vi "attribute_get_cache_or_default_value.vi"(7 "Attribute":T1={"Identifier"="", "Descriptive name"="", "Data Type"=enum."Integer 32", "Command"="", "Access"=2, "Range Table"="", "Read Callback"="", "Write Callback"="", "Range Callback"="", "Check Callback"="", "Rngtable Callback"="", "Coerce Callback"="", "Supported Models"="", "Instrument Options"="", "Repeated Capabilities"="", "Check Status Callback"="", "Index"=0, "Flag: OPC Wait"=FALSE, "Flag: Dont check status"=FALSE, "Flag: Cache Only"=FALSE} {"Access" items=["Read Only", "Write Only", "Read/Write"]}, 8 "error in":errorcluster, 11 "VISA resource name":refnum<visa-resource-name>) -> (0 "error out":errorcluster, 1 "Integer 32 out":i32, 2 "Double out":dbl, 3 "VISA resource name out":refnum<visa-resource-name>, 4 "String out":string, 5 "Integer 64 out":i64, 6 "Boolean out":bool, 9 "Exists in cache":bool)   [LabVIEW 2014, in "rszvl_rsidr_core.lvlib"]
uses:
  rszvl_rsidr_core.lvlib
  type_Attribute.ctl
  type_Attribute_Data_Type.ctl
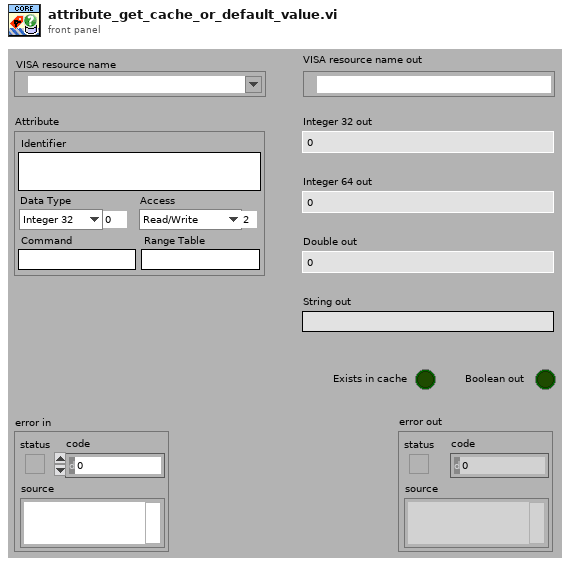
[diagram p1: front panel]
types:
  T1 = typedef "rszvl_rsidr_core.lvlib/type_Attribute.ctl" = cluster{"Identifier":string, "Descriptive name":string, "Data Type":T2, "Command":string, "Access":u16, "Range Table":string, "Read Callback":string, "Write Callback":string, "Range Callback":string, "Check Callback":string, "Rngtable Callback":string, "Coerce Callback":string, "Supported Models":string, "Instrument Options":string, "Repeated Capabilities":string, "Check Status Callback":string, "Index":i32, "Flag: OPC Wait":bool, "Flag: Dont check status":bool, "Flag: Cache Only":bool}
  T2 = typedef "rszvl_rsidr_core.lvlib/type_Attribute_Data_Type.ctl" = enum16{"Integer 32", "Double", "String", "Boolean", "None", "Integer 64"}
  T3 = enum16{"Initialize", "Check", "Get Numeric Value", "Get Default Value"}
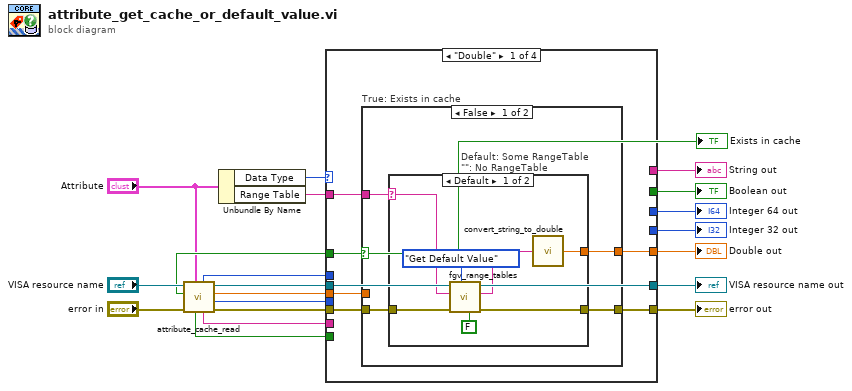
[diagram p0: block diagram]
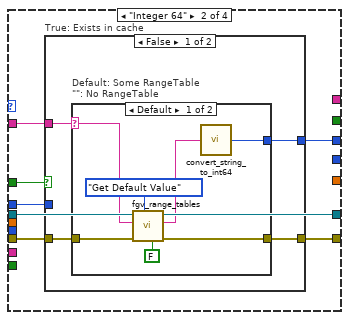
[diagram p4: hidden frame]
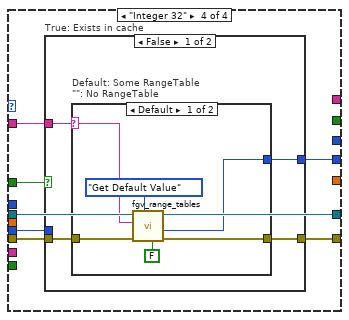
[diagram p8: hidden frame]
diagram:
  n1 = call "attribute_cache_read.vi"("Attribute"="Attribute", "error in"="error in", "VISA resource name"="VISA resource name") -> ("error out"=w12:errorcluster, "Integer 32 out"=w6:i32, "Double out"=w9:dbl, "VISA resource name out"=w11:refnum<visa-resource-name>, "String out"=w5:string, "Integer 64 out"=w8:i64, "Boolean out"=w3:bool, "Exists in cache"=w10:bool)  [unwired: 1 in]
  "Exists in cache" <- w10
  n2 = Unbundle By Name("Attribute") -> ("Data Type"=w17:T2, "Range Table"=w7:string)
  n3 = case shown="\"Double\"" w17 {
    tunnel: w12 -> [w24 w43 w66 w69]
    tunnel: w11 -> [w25 w44 w65 w70]
    tunnel: [w27 w48 w66 w73] -> w20
    tunnel: [w25 w44 w65 w70] -> w19
    tunnel: [w26 _ _ _] -> w18
    tunnel: [_ _ _ w72] -> w16
    tunnel: [_ w47 _ _] -> w15
    tunnel: w10 -> [w22 w45 _ w67]
    tunnel: w9 -> [w23 _ _ _]
    tunnel: w8 -> [_ w46 _ _]
    tunnel: w7 -> [w21 w42 _ w71]
    tunnel: w6 -> [_ _ _ w68]
    tunnel: w5 -> [_ _ w64 _]
    tunnel: [_ _ w64 _] -> w4
    tunnel: w3 -> [_ _ w63 _]
    tunnel: [_ _ w63 _] -> w2
    frame "Double" {
      n4 = case "True: Exists in cache" shown="False" w22 {
        tunnel: w24 -> [w30 w41]
        tunnel: w23 -> [_ w40]
        tunnel: [w29 w41] -> w27
        tunnel: w21 -> [w31 _]
        tunnel: [w28 w40] -> w26
        frame False {
          n5 = case "Default: Some RangeTable\n\"\": No RangeTable" shown="Default" w31 {
            selector: w31 -> [w35 _]
            tunnel: w30 -> [w38 w39]
            tunnel: [w37 w39] -> w29
            tunnel: [w33 _] -> w28
            frame Default {
              n6 = call "fgv_range_tables.vi"("Range Checking"=FALSE, "Operation"=T3."Get Default Value", "error in"=w38, "Range Table ID in"=w35) -> ("error out"=w37:errorcluster, "Default value out"=w32:string)  [unwired: 4 in, 2 out]
              n7 = call "convert_string_to_double.vi"("String in"=w32) -> ("double value out"=w33:dbl)  [unwired: 4 in]
            }
            frame "" {
            }
          }
        }
        frame True {
        }
      }
    }
    frame "Integer 64" {
      n8 = case "True: Exists in cache" shown="False" w45 {
        tunnel: w43 -> [w51 w62]
        tunnel: w46 -> [_ w61]
        tunnel: [w50 w62] -> w48
        tunnel: w42 -> [w52 _]
        tunnel: [w49 w61] -> w47
        frame False {
          n9 = case "Default: Some RangeTable\n\"\": No RangeTable" shown="Default" w52 {
            selector: w52 -> [w56 _]
            tunnel: w51 -> [w59 w60]
            tunnel: [w58 w60] -> w50
            tunnel: [w54 _] -> w49
            frame Default {
              n10 = call "fgv_range_tables.vi"("Range Checking"=FALSE, "Operation"=T3."Get Default Value", "error in"=w59, "Range Table ID in"=w56) -> ("error out"=w58:errorcluster, "Default value out"=w53:string)  [unwired: 4 in, 2 out]
              n11 = call "convert_string_to_int64.vi"("String in"=w53) -> ("int64 value out"=w54:i64)  [unwired: 4 in]
            }
            frame "" {
            }
          }
        }
        frame True {
        }
      }
    }
    frame Default {
    }
    frame "Integer 32" {
      n12 = case "True: Exists in cache" shown="False" w67 {
        tunnel: w69 -> [w77 w86]
        tunnel: w68 -> [_ w85]
        tunnel: [w76 w86] -> w73
        tunnel: [w75 w85] -> w72
        tunnel: w71 -> [w74 _]
        frame False {
          n13 = case "Default: Some RangeTable\n\"\": No RangeTable" shown="Default" w74 {
            selector: w74 -> [w80 _]
            tunnel: w77 -> [w83 w84]
            tunnel: [w82 w84] -> w76
            tunnel: [w78 _] -> w75
            frame Default {
              n14 = call "fgv_range_tables.vi"("Range Checking"=FALSE, "Operation"=T3."Get Default Value", "error in"=w83, "Range Table ID in"=w80) -> ("error out"=w82:errorcluster, "Numeric I32 Value out"=w78:i32)  [unwired: 4 in, 2 out]
            }
            frame "" {
            }
          }
        }
        frame True {
        }
      }
    }
  }
  "VISA resource name out" <- w19
  "error out" <- w20
  "Integer 64 out" <- w15
  "Integer 32 out" <- w16
  "Double out" <- w18
  "String out" <- w4
  "Boolean out" <- w2
